vi "ConnectionInfo.vi"(8 "error in (no error)":errorcluster, 11 "AdsNET in":refnum<class "AdsNET.lvclass">) -> (0 "error out":errorcluster, 2 "ConnectionInfo":T1, 3 "AdsNET out":refnum<class "AdsNET.lvclass">)   [LabVIEW 2016, in "TCatAdsNet.lvlib" / "AdsNET.lvclass"]
doc: "Get ADS connection infos for Client and Server."
uses:
  AdsNET.lvclass
  AdsNET.lvclass/AdsNET.ctl
  C:/Users/Maurizio/Projects/twincat-lv-ads-library/TCatAdsNet Library/TwinCAT.Ads.dll
  TwinCAT.Ads.dll
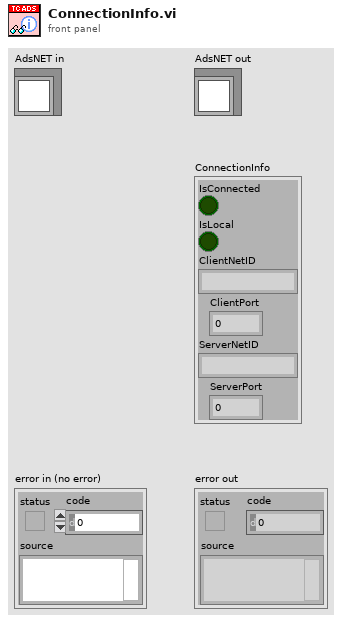
[diagram p1: front panel]
types:
  T1 = cluster{"IsConnected":bool, "IsLocal":bool, "ClientNetID":string, "ClientPort":i32, "ServerNetID":string, "ServerPort":i32}
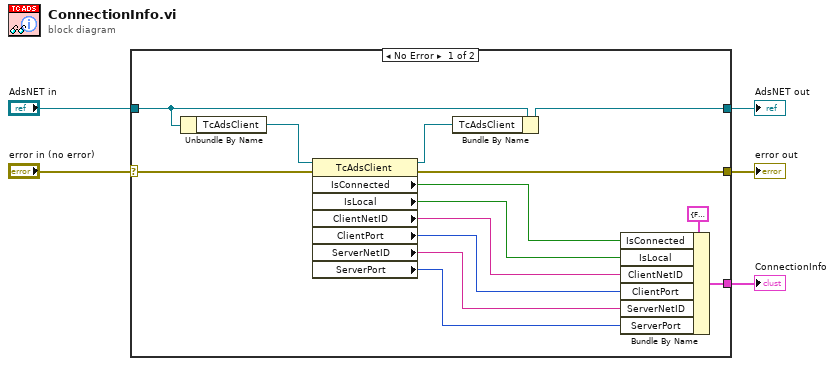
[diagram p0: block diagram]
diagram:
  n1 = case shown="No Error" "error in (no error)" {
    selector: "error in (no error)" -> [w9 w21]
    tunnel: [w8 w21] -> w4
    tunnel: [w7 w20] -> w2
    tunnel: "AdsNET in" -> [w19 w20]
    tunnel: [w14 _] -> w1
    frame No Error {
      n2 = Unbundle By Name(w19) -> ("TcAdsClient"=w18:refnum<k24>)
      n3 = property class="TcAdsClient"(reference=w18, error in=w9) -> (reference out=w6:refnum<k24>, error out=w8:errorcluster, "IsConnected"=w16:bool, "IsLocal"=w15:bool, "ClientNetID"=w13:string, "ClientPort"=w12:i32, "ServerNetID"=w11:string, "ServerPort"=w10:i32)
      n4 = Bundle By Name(cluster=w19, "TcAdsClient"=w6) -> (w7:refnum<class "AdsNET.lvclass">)
      n5 = Bundle By Name(cluster=T1 {"IsConnected"=FALSE, "IsLocal"=FALSE, "ClientNetID"="", "ClientPort"=0, "ServerNetID"="", "ServerPort"=0}, "IsConnected"=w16, "IsLocal"=w15, "ClientNetID"=w13, "ClientPort"=w12, "ServerNetID"=w11, "ServerPort"=w10) -> (w14:T1)
    }
    frame Error {
    }
  }
  "error out" <- w4
  "AdsNET out" <- w2
  "ConnectionInfo" <- w1
